vi "Set Dialog UI Ref.vi"(8 "error in (no error)":errorcluster, 10 "Main ctls and VI ref":T1, 11 "ScriptDialog in":refnum<class "ScriptDialog.lvclass">) -> (0 "error out":errorcluster, 3 "ScriptDialog out":refnum<class "ScriptDialog.lvclass">)   [LabVIEW 2015, in "ScriptDialog.lvclass"]
uses:
  ScriptDialog.lvclass
  Type Definitiions/Dialog Main ctls and VI ref.ctl
  ScriptDialog.lvclass/ScriptDialog.ctl
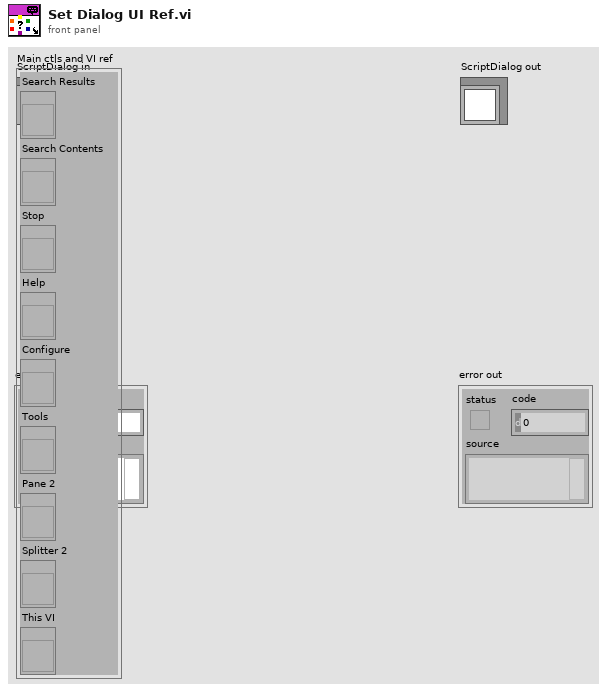
[diagram p1: front panel]
types:
  T1 = typedef "ScriptDialog.lvclass/Dialog Main ctls and VI ref.ctl" = cluster{"Search Results":refnum<vi>, "Search Contents":refnum<vi>, "Stop":refnum<vi>, "Help":refnum<vi>, "Configure":refnum<vi>, "Tools ":refnum<vi>, "Pane 2":refnum<vi>, "Splitter 2":refnum<vi>, "This VI":refnum<vi>}
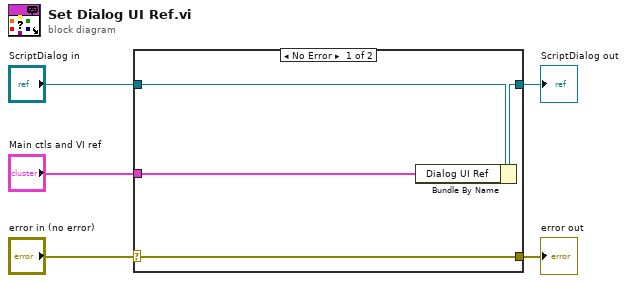
[diagram p0: block diagram]
diagram:
  n1 = case shown="No Error" "error in (no error)" {
    selector: "error in (no error)" -> [w9 w10]
    tunnel: [w9 w10] -> w4
    tunnel: [w7 w11] -> w2
    tunnel: "ScriptDialog in" -> [w8 w11]
    tunnel: "Main ctls and VI ref" -> [w6 _]
    frame No Error {
      n2 = Bundle By Name(cluster=w8, "Dialog UI Ref"=w6) -> (w7:refnum<class "ScriptDialog.lvclass">)
    }
    frame Error {
    }
  }
  "error out" <- w4
  "ScriptDialog out" <- w2
